vi "AM.vi"() -> ()   [LabVIEW 2013]
uses:
  <vilib>/sound2/lvsound2.llb/Sound Data Format.ctl
  <vilib>/Analysis/2dsp.llb/Rational Resample (single channel, DBL).vi
  <vilib>/sound2/lvsound2.llb/Sound Output Write (DBL).vi
  <vilib>/express/express analysis/Spectral/Block/exnSpectralBlock spectral measurements RMS poly.vi
  <vilib>/express/express analysis/Spectral/Block/exnSpectralBlock spectral measurements RMS WFM.vi
  <vilib>/express/express analysis/Spectral/XNode/ExpressSpectralMeasurementsBlockNode.xnode
  rtlsdr/rtlsdr.lvlib
  <vilib>/Analysis/NI_AALPro.lvlib
panel:
  in  "Device index":u32=1
  out "Samples Acquired":u32
  out "# elements in queue":i32
  out "DevRefnum":u64
  out "Spectrum (FFT)":cluster{"f0":dbl, "df":dbl, "magnitude":dbl[]}(graph)
  out "XY Graph":cluster{dbl[], dbl[]}(graph)
  out "error out":errorcluster
  in  "sound format":T1={"sample rate (S/s)"=44100.0, "number of channels"=1, "bits per sample"=16}
  in  "stop":bool
  in  "Center frequency":u32=422495000
  in  "IQ rate":u32=1000000
  out "error out":errorcluster
  # "FM Receiver"
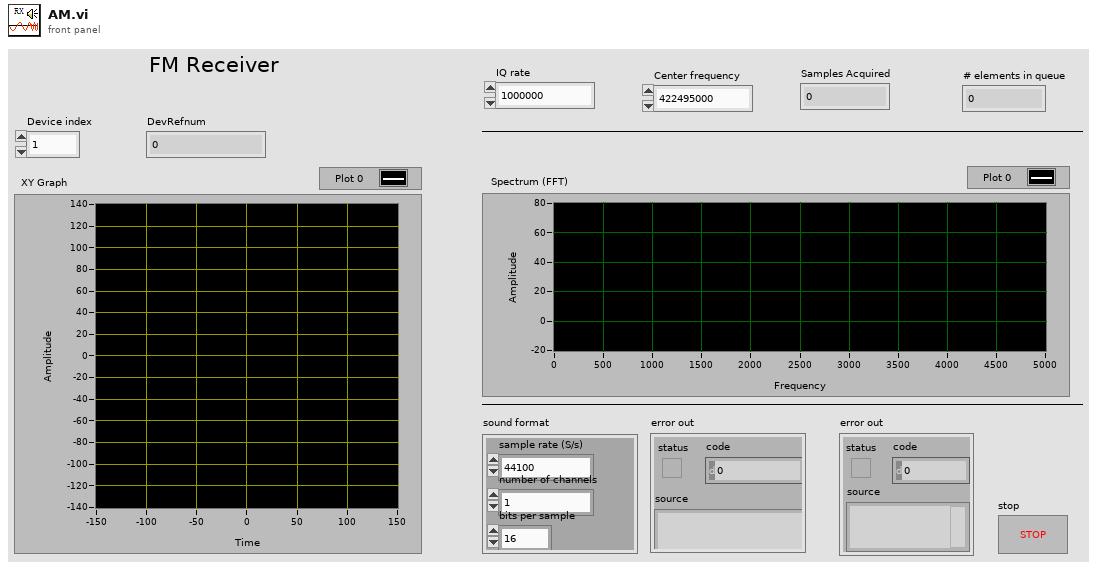
[diagram p1: front panel]
types:
  T1 = typedef "Sound Data Format.ctl" = cluster{"sample rate (S/s)":dbl, "number of channels":i32, "bits per sample":i32}
  T2 = typedef "Sound Output Task ID.ctl" = u32
  T3 = cluster{"averaging mode":u16, "weighting mode":u16, "number of averages":u32}
  T4 = cluster{"dB On (F)":bool, "unwrap phase (F)":bool, "convert to degree (F)":bool}
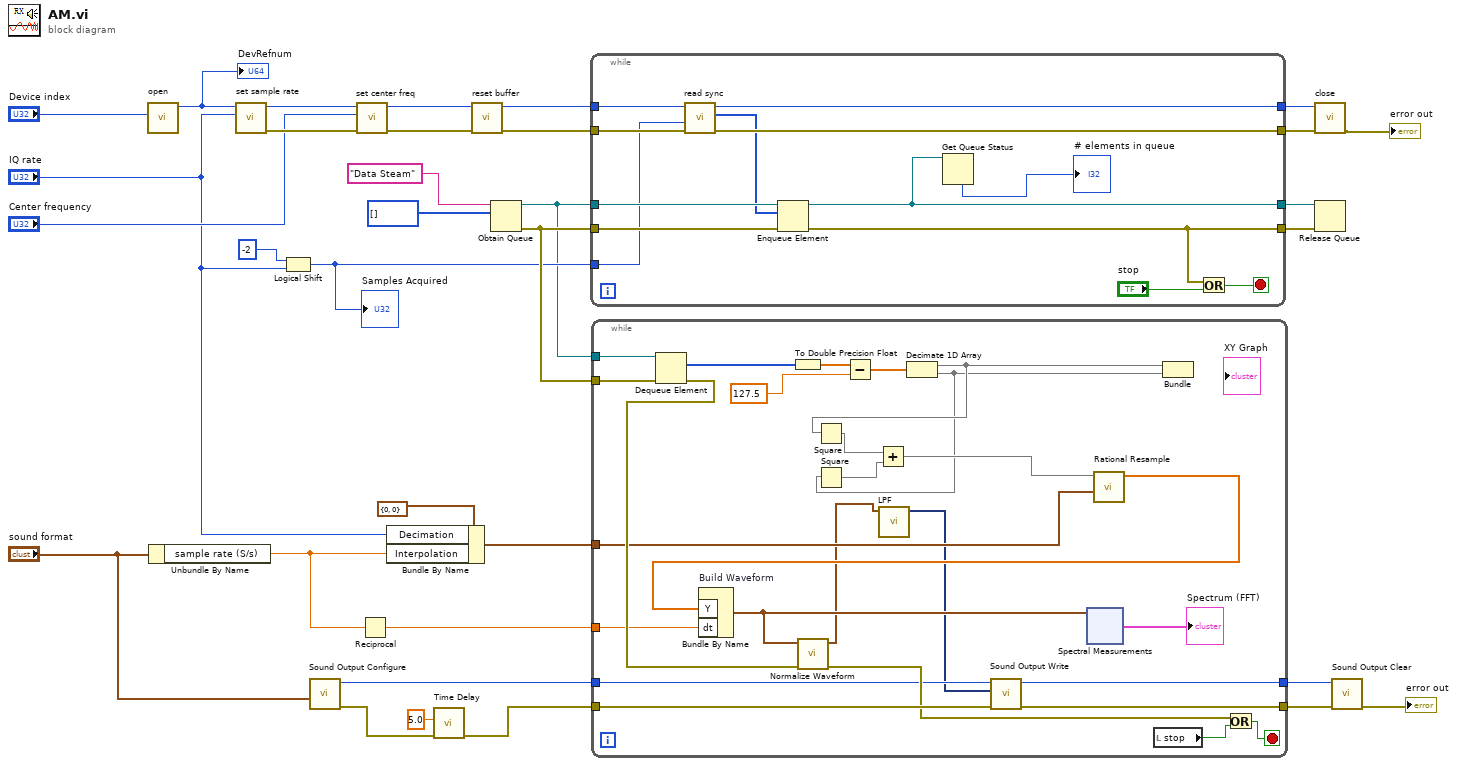
[diagram p0: block diagram]
diagram:
  n1 = call "open.vi"("index"="Device index") -> ("DevRefnum"=w26:u64)  [unwired: 9 in, 1 out]
  "DevRefnum" <- w26
  n2 = Unbundle By Name("sound format") -> ("sample rate (S/s)"=w1:dbl)
  n3 = call "set sample rate.vi"("rate"="IQ rate", "DevRefnum"=w26) -> ("error out"=w28:errorcluster, "DevRefnum"=w30:u64)  [unwired: 7 in, 1 out]
  n4 = Logical Shift(y=i16 -2, x="IQ rate") -> (x << y=w3:u32)
  "Samples Acquired" <- w3
  n5 = call <vilib>:"Sound Output Configure.vi"("sound format"="sound format") -> ("error out"=w8:errorcluster, "task ID"=w18:T2)  [unwired: 9 in]
  n6 = call "set center freq.vi"("error in (no error)"=w28, "freq"="Center frequency", "DevRefnum"=w30) -> ("error out"=w27:errorcluster, "DevRefnum"=w29:u64)  [unwired: 6 in, 1 out]
  n7 = Reciprocal(x=w1) -> (1/x=w11:dbl)
  n8 = Bundle By Name(cluster=cluster{"Interpolation":i32, "Decimation":i32} {"Interpolation"=0, "Decimation"=0}, "Decimation"="IQ rate", "Interpolation"=w1) -> (w10:cluster{"Interpolation":i32, "Decimation":i32})
  n9 = call "Time Delay"("error in (no error)"=w8, "Delay Time (s)"=5.0) -> ("error out"=w9:errorcluster)  [unwired: 9 in]
  n10 = call "reset buffer.vi"("error in (no error)"=w27, "DevRefnum"=w29) -> ("error out"=w23:errorcluster, "DevRefnum"=w24:u64)  [unwired: 8 in]
  n11 = Obtain Queue(name (unnamed)="Data Steam", element data type=u8[] [] ("buf 2")) -> (queue out=w2:refnum<queue>, error out=w4:errorcluster)  [unwired: 3 in, 1 out]
  n12 = while {
    tunnel: [w44] -> w21
    tunnel: w24 -> [w46]
    tunnel: w23 -> [w45]
    tunnel: [w43] -> w20
    tunnel: w3 -> [w34]
    tunnel: w2 -> [w41]
    tunnel: [w40] -> w14
    tunnel: w4 -> [w39]
    tunnel: [w37] -> w13
    stop <- w35 stop-if-true
    n13 = call "read sync.vi"("error in (no error)"=w45, "len"=w34, "DevRefnum"=w46) -> ("error out"=w43:errorcluster, "buf 2"=w38:u8[], "DevRefnum"=w44:u64)  [unwired: 6 in]
    n14 = Enqueue Element(queue=w41, element=w38, error in (no error)=w39) -> (queue out=w40:refnum<queue>, error out=w37:errorcluster)  [unwired: 1 in, 1 out]
    n15 = Get Queue Status(queue=w40) -> (# elements in queue=→"# elements in queue":i32)  [unwired: 2 in, 7 out]
    n16 = Or(x=w37, y="stop") -> (x .or. y?=w35:bool)
  }
  n17 = while {
    tunnel: w18 -> [w56]
    tunnel: [w67] -> w17
    tunnel: [w66] -> w16
    tunnel: w9 -> [w68]
    tunnel: w2 -> [w65]
    tunnel: w11 -> [w57]
    tunnel: w10 -> [w58]
    tunnel: w4 -> [w63]
    stop <- w59 stop-if-true
    n18 = Dequeue Element(queue=w65, error in (no error)=w63) -> (element=w64:u8[], error out=w62:errorcluster)  [unwired: 1 in, 2 out]
    n19 = To Double Precision Float(number=w64) -> (double precision float=w71:dbl[])
    n20 = Subtract(x=w71, y=127.5) -> (x-y=w69:dbl[])
    n21 = Decimate 1D Array "Decimate 1D Array"(w69) -> (w50:dbl[], w49:dbl[])
    n22 = Square(x=w50) -> (x^2=w53:dbl[])
    n23 = Square(x=w49) -> (x^2=w52:dbl[])
    n24 = Add(x=w53, y=w52) -> (x+y=w51:dbl[])
    n25 = call-poly <vilib>:"Rational Resample.vi"("resample factor"=w58, "X"=w51) -> ("Y"=w72:dbl[])  [unwired: 7 in, 2 out]
    n26 = Bundle By Name "Build Waveform"("Y"=w72, "dt"=w57) -> (w55:waveform(dbl))  [unwired: 1 in]
    n27 = call <vilib>:"Normalize Waveform.vi"("error in (no error)"=w62, "waveform in"=w55) -> ("error out"=w61:errorcluster, "normalized waveform"=w48:waveform(dbl))  [unwired: 6 in, 2 out]
    n28 = call "LPF"("Signal"=w48) -> ("Filtered Signal"=w47:dynamicdata)  [unwired: 9 in, 1 out]
    n29 = call-poly <vilib>:"Sound Output Write.vi"("error in (no error)"=w68, "data"=w47, "task ID"=w56) -> ("error out"=w66:errorcluster, "task ID out"=w67:T2)  [unwired: 7 in]
    n30 = xnode ("Spectral Measurements")("Signals"=w55) -> ("FFT - (RMS)"=→"Spectrum (FFT)":cluster{"f0":dbl, "df":dbl, "magnitude":dbl[]})  [unwired: 1 in, 2 out]
    n31 = local read "stop"() -> (w60:bool)
    n32 = Bundle(w50, w49) -> ()  [unwired: 1 in, 1 out]
    n33 = Or(x=w61, y=w60) -> (x .or. y?=w59:bool)
  }
  n34 = call "close.vi"("error in (no error)"=w20, "DevRefnum"=w21) -> ("error out"=→"error out":errorcluster)  [unwired: 8 in, 1 out]
  n35 = Release Queue(queue=w14, error in (no error)=w13) -> ()  [unwired: 1 in, 3 out]
  n36 = call <vilib>:"Sound Output Clear.vi"("error in (no error)"=w16, "task ID"=w17) -> ("error out"=→"error out":errorcluster)  [unwired: 9 in]
